vi "Configure Power Offset.vi"(8 "error in (no error)":errorcluster, 10 "Power Offset":dbl, 11 "PM-EMP in":refnum<class "PM-EMP.lvclass">) -> (0 "error out":errorcluster, 3 "PM-EMP out":refnum<class "PM-EMP.lvclass">)   [LabVIEW 2020, in "PM-EMP.lvclass"]
uses:
  PM-EMP.lvclass
  C:/Sandbox/Git_Sandbox/WiSpry Test Framework source code (LV20)/WiSpry Test Framework/Instruments/Instrument.lvclass
  Instrument.lvclass/Instrument.ctl
  Instrument.lvclass
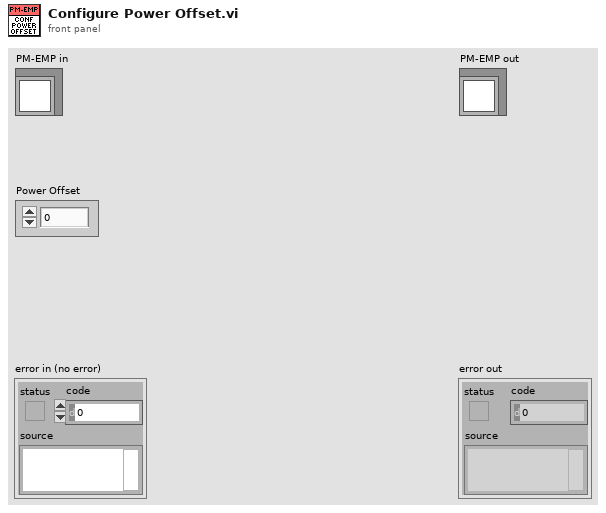
[diagram p1: front panel]
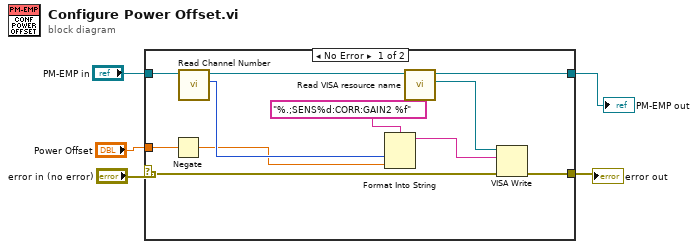
[diagram p0: block diagram]
diagram:
  n1 = case shown="No Error" "error in (no error)" {
    selector: "error in (no error)" -> [w16 w17]
    tunnel: "PM-EMP in" -> [w10 w18]
    tunnel: "Power Offset" -> [w7 _]
    tunnel: [w12 w17] -> w2
    tunnel: [w11 w18] -> w1
    frame No Error {
      n2 = Negate(x=w7) -> (-x=w6:dbl)
      n3 = call-dynamic "Read Channel Number.vi"("Power Meter in"=w10) -> ("Channel Number"=w8:u8, "Power Meter out"=w9:refnum<class "PM-EMP.lvclass">)  [unwired: 9 in]
      n4 = Format Into String(format string="%.;SENS%d:CORR:GAIN2 %f", w8, w6) -> (resulting string=w13:string)  [unwired: 2 in, 1 out]
      n5 = call "Read VISA resource name.vi"("Instrument in"=w9) -> ("VISA resource name"=w15:refnum<visa-resource-name>, "Instrument out"=w11:refnum<class "PM-EMP.lvclass">)  [unwired: 9 in]
      n6 = VISA Write(VISA resource name=w15, write buffer=w13, error in (no error)=w16) -> (error out=w12:errorcluster)  [unwired: 2 out]
    }
    frame Error {
    }
  }
  "error out" <- w2
  "PM-EMP out" <- w1
